vi "Get Connections.vi"(6 "instrument type id":string, 8 "error in":errorcluster, 9 "sites":i32[](array[numeric]), 10 "pin or relay names":string[](array[string]), 11 "connection map in":refnum<class "Connection Map.lvclass">) -> (0 "error out":errorcluster, 1 "pin or relay names found":string[](array[string]), 2 "connections":T1[](array[typedef]), 3 "connection map out":refnum<class "Connection Map.lvclass">)   [LabVIEW 2020, in "NI Session Management V1 Client.lvlib" / "Connection Map.lvclass"]
uses:
  Connection Map.lvclass
  Session Reservation/Connection with Session.ctl
  Session Reservation/Connection.ctl
  Connection Map.lvclass/Connection Map.ctl
  e459d0b4-a487-43d8-9fc7-6ae275c711c2.vi
  Session Reservation/Session Reservation.lvclass
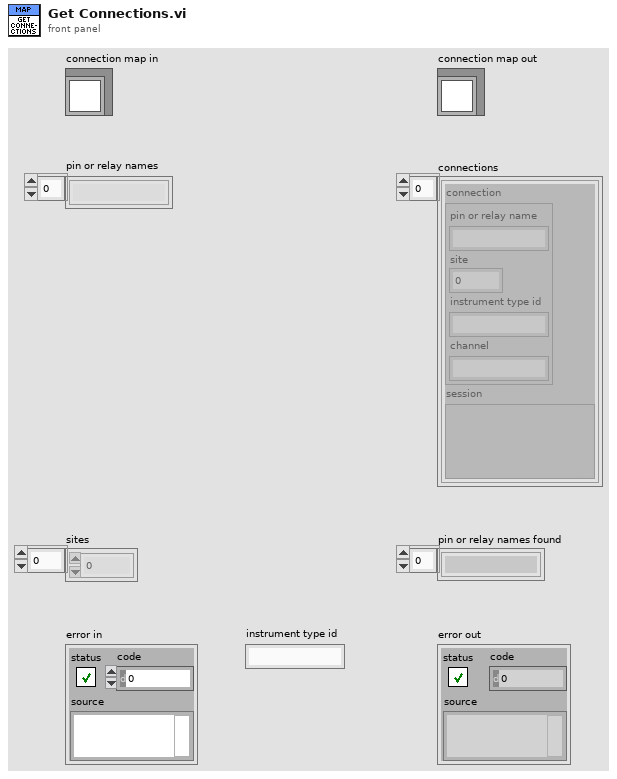
[diagram p1: front panel]
types:
  T1 = typedef "NI Session Management V1 Client.lvlib/Session Reservation.lvclass/Connection with Session.ctl" = cluster{"connection":T2, "session":variant}
  T2 = typedef "NI Session Management V1 Client.lvlib/Session Reservation.lvclass/Connection.ctl" = cluster{"pin or relay name":string, "site":i32, "instrument type id":string, "channel":string}
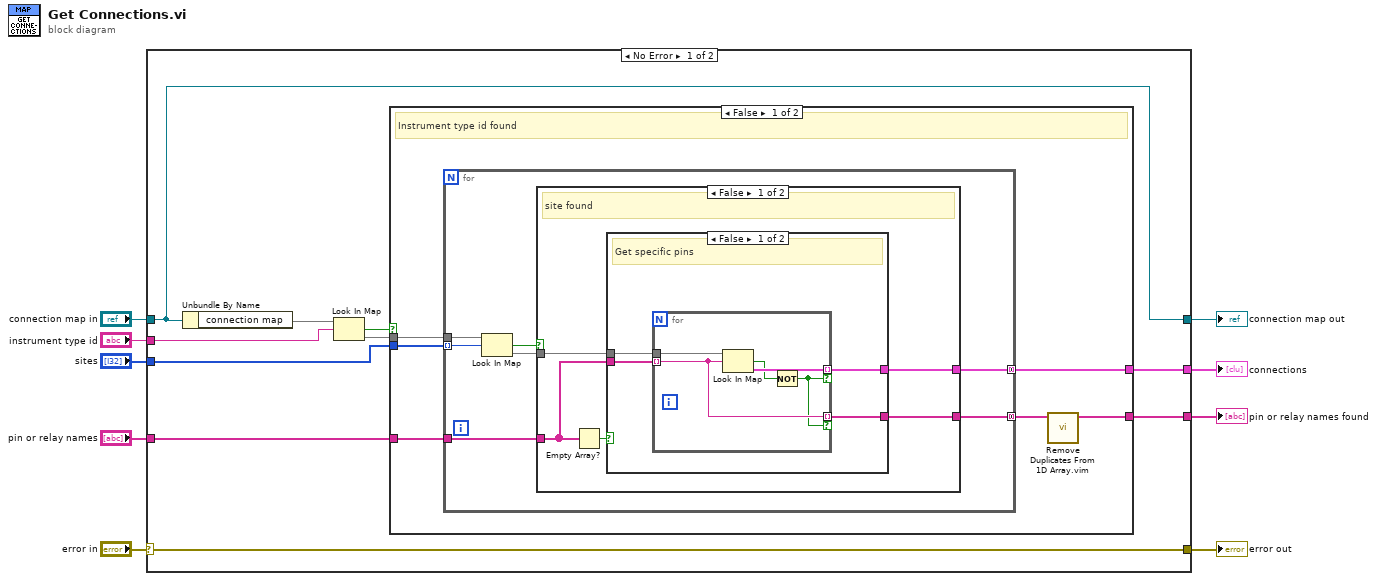
[diagram p0: block diagram]
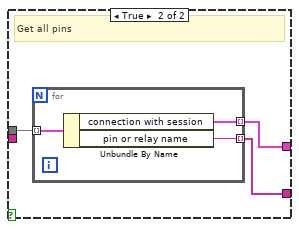
[diagram p2: hidden frame]
diagram:
  n1 = case shown="No Error" "error in" {
    selector: "error in" -> [w11 w54]
    tunnel: [w11 w54] -> w8
    tunnel: [w15 w53] -> w6
    tunnel: "connection map in" -> [w15 w53]
    tunnel: "instrument type id" -> [w13 _]
    tunnel: "sites" -> [w17 _]
    tunnel: "pin or relay names" -> [w16 _]
    tunnel: [w12 _] -> w2
    tunnel: [w10 _] -> w1
    frame No Error {
      n2 = Unbundle By Name(w15) -> ("connection map"=w14:map{string, map{i32, map{string, T1}}})
      n3 = Look In Map(map=w14, key=w13) -> (key not found?=w18:bool, value=w19:map{i32, map{string, T1}})  [unwired: 1 in]
      n4 = case shown="False" w18 {
        tunnel: w19 -> [w25 _]
        tunnel: w17 -> [w24 _]
        tunnel: w16 -> [w23 _]
        tunnel: [w22 _] -> w12
        tunnel: [w20 _] -> w10
        frame False {
          # "Instrument type id found"
          n5 = for {
            tunnel: w25 -> [w32]
            tunnel: w24 -> [w26] mode=indexing
            tunnel: w23 -> [w29]
            tunnel: [w28] -> w22 mode=concatenating
            tunnel: [w27] -> w21 mode=concatenating
            n6 = Look In Map(map=w32, key=w26) -> (key not found?=w31:bool, value=w30:map{string, T1})  [unwired: 1 in]
            n7 = case shown="False" w31 {
              tunnel: w30 -> [w37 _]
              tunnel: w29 -> [w35 _]
              tunnel: [w36 _] -> w28
              tunnel: [w33 _] -> w27
              frame False {
                # "site found"
                n8 = Empty Array?(array=w35) -> (empty?=w34:bool)
                n9 = case shown="False" w34 {
                  tunnel: w37 -> [w41 w49]
                  tunnel: [w39 w48] -> w36
                  tunnel: w35 -> [w40 _]
                  tunnel: [w38 w47] -> w33
                  frame False {
                    # "Get specific pins"
                    n10 = for {
                      tunnel: w41 -> [w46]
                      tunnel: w40 -> [w43] mode=indexing
                      tunnel: [w45] -> w39 mode=indexing if=w42
                      tunnel: [w43] -> w38 mode=indexing if=w42
                      n11 = Look In Map(map=w46, key=w43) -> (key not found?=w44:bool, value=w45:T1)  [unwired: 1 in]
                      n12 = Not(x=w44) -> (.not. x?=w42:bool)
                    }
                  }
                  frame True {
                    # "Get all pins"
                    n13 = for {
                      tunnel: w49 -> [w52] mode=indexing
                      tunnel: [w51] -> w48 mode=indexing
                      tunnel: [w50] -> w47 mode=indexing
                      n14 = Unbundle By Name(w52) -> ("connection with session"=w51:T1, "pin or relay name"=w50:string)
                    }
                  }
                }
              }
              frame True {
                # "site not found"
              }
            }
          }
          n15 = call "Remove Duplicates From 1D Array.vim"("array"=w21) -> ("array with duplicates removed"=w20:string[])  [unwired: 10 in]
        }
        frame True {
          # "Instrument type id not found"
        }
      }
    }
    frame Error {
    }
  }
  "error out" <- w8
  "connection map out" <- w6
  "connections" <- w2
  "pin or relay names found" <- w1
